vi "comm lock2.vi"(8 "error in (no error)":errorcluster, 10 "Timeout (-1:infinitive)":i32=-1, 11 "Comm Handle":u32) -> (0 "error out":errorcluster, 1 "Locked?":bool, 3 "dup Comm Handle":u32)   [LabVIEW 2017, in "lvserial.lvlib"]
doc: "Locks the serial port."
uses:
  lvserial.lvlib
  lvserial.dll
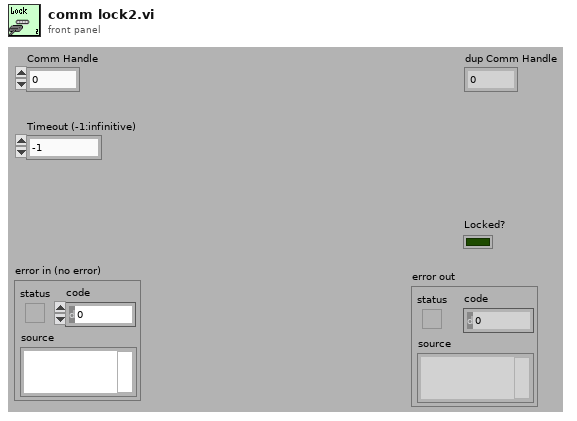
[diagram p1: front panel]
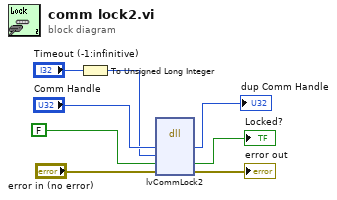
[diagram p0: block diagram]
diagram:
  n1 = To Unsigned Long Integer(number="Timeout (-1:infinitive)") -> (unsigned 32bit integer=w5:u32)
  n2 = dll-call lib="lvserial.dll" fn="lvCommLock2"("hComm"="Comm Handle", "ulTimeout"=w5, "Locked?"=FALSE, "error in (no error)"="error in (no error)") -> ("hComm"=→"dup Comm Handle":u32, "Locked?"=→"Locked?":bool, "error in (no error)"=→"error out":errorcluster)  [unwired: 4 in, 3 out]
